vi "Get In ProgramData.vi"(7 "System Path Only (F)":bool, 10 "error in (no error)":errorcluster) -> (2 "error out":errorcluster, 3 "Path":path)   [LabVIEW 2021, in "Path Utilities.lvlib"]
doc: "Returns ProgramData path appended with base path.\neg: \"C:\\ProgramData\\Base\\Path\"\n\nIf \"System Path Only\" is True, returns only ProgramFiles path.\n\"C:\\ProgramData\"\n\nUse \"Set Base Path.vi\" to set the base path for this vi."
uses:
  Path Utilities.lvlib
  TypeDefs/FGV State.ctl
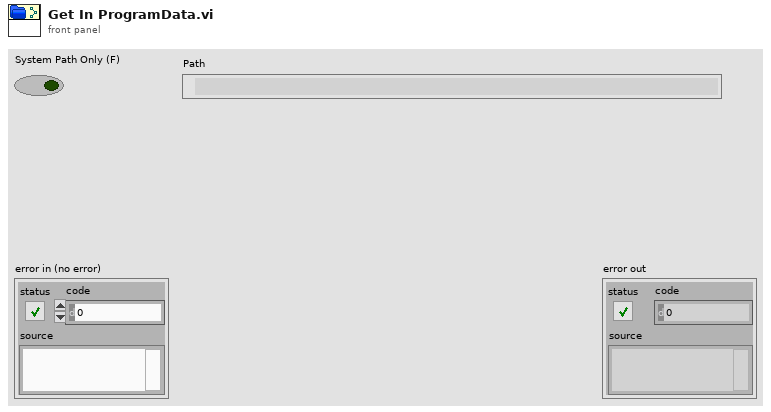
[diagram p1: front panel]
types:
  T1 = typedef "Path Utilities.lvlib/FGV State.ctl" = enum16{"Set Base Path", "Get Program Files", "Get Program Data", "Get App Data Local", "Get App Data Roaming", "Get User Documents", "Get Public Documents"}
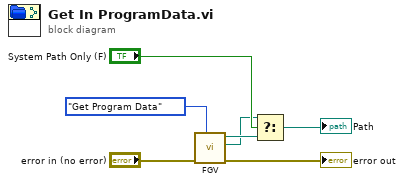
[diagram p0: block diagram]
diagram:
  n1 = call "FGV.vi"("FGV State"=FGV_State."Get Program Data", "error in (no error)"="error in (no error)") -> ("error out"=→"error out":errorcluster, "System Directory Out"=w1:path, "Path Out"=w3:path)  [unwired: 7 in]
  n2 = Select(t=w1, s="System Path Only (F)", f=w3) -> (s? t:f=→"Path":path)
